vi "SendEmail.vi"(0 "To Address":string="kchambe1@nd.edu", 1 "To DisplayName":string="Karen Ostdiek ", 2 "Path to File":path=path "C:/Users/Public/Documents/AMS_VIs/2015/Karen/textfile", 3 "Subject":string, 4 "Body":string) -> ()   [LabVIEW 2014]
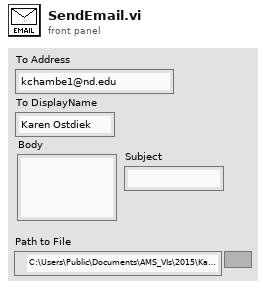
[diagram p1: front panel]
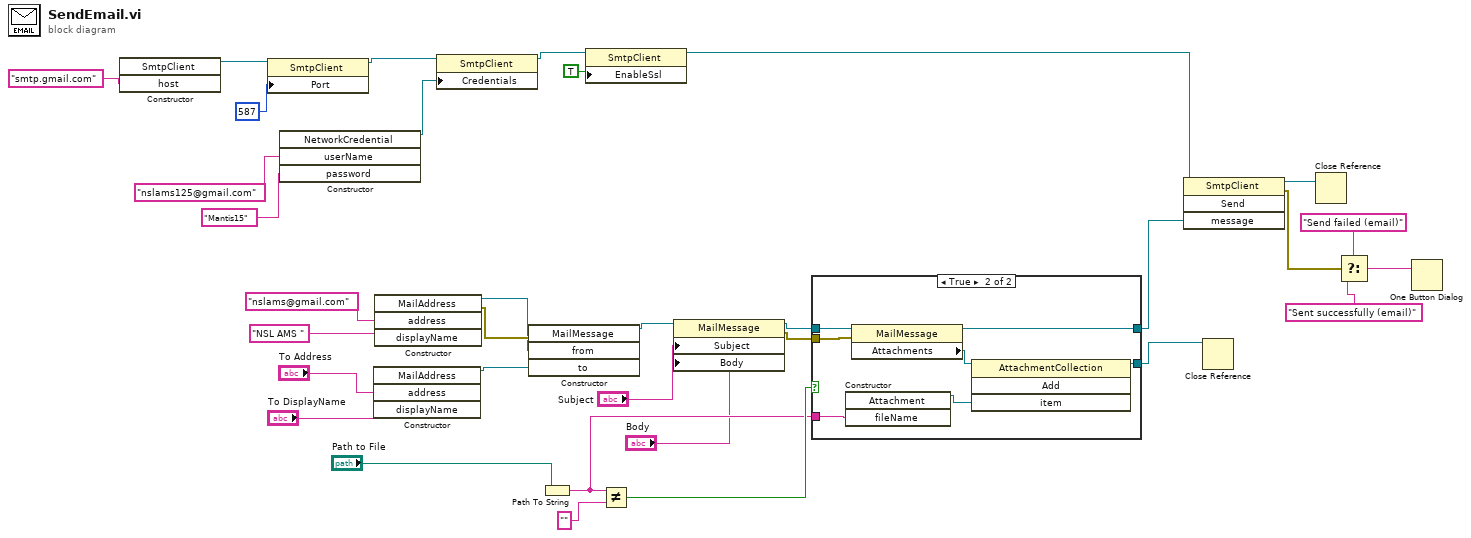
[diagram p0: block diagram]
diagram:
  n1 = constructor class="SmtpClient"("host"="smtp.gmail.com") -> (reference out=w32:refnum<k24>)  [unwired: 3 in, 3 out]
  n2 = property class="SmtpClient"(reference=w32, "Port"=587) -> (reference out=w30:refnum<k24>)  [unwired: 1 in, 1 out]
  n3 = constructor class="NetworkCredential"("userName"="nslams125@gmail.com", "password"="Mantis15") -> (reference out=w27:refnum<k24>)  [unwired: 3 in, 4 out]
  n4 = constructor class="MailAddress"("address"="To Address", "displayName"="To DisplayName") -> (reference out=w17:refnum<k24>)  [unwired: 3 in, 4 out]
  n5 = constructor class="MailAddress"("address"="nslams@gmail.com", "displayName"="NSL AMS ") -> (reference out=w18:refnum<k24>, error out=w19:errorcluster)  [unwired: 3 in, 3 out]
  n6 = property class="SmtpClient"(reference=w30, "Credentials"=w27) -> (reference out=w26:refnum<k24>)  [unwired: 1 in, 1 out]
  n7 = constructor class="MailMessage"(error in=w19, "from"=w18, "to"=w17) -> (reference out=w16:refnum<k24>)  [unwired: 2 in, 4 out]
  n8 = Path To String(path="Path to File") -> (string=w10:string)
  n9 = property class="SmtpClient"(reference=w26, "EnableSsl"=TRUE) -> (reference out=w25:refnum<k24>)  [unwired: 1 in, 1 out]
  n10 = Not Equal?(x=w10, y="") -> (x != y?=w13:bool)
  n11 = property class="MailMessage"(reference=w16, "Subject"="Subject", "Body"="Body") -> (reference out=w12:refnum<k24>, error out=w11:errorcluster)  [unwired: 1 in]
  n12 = case shown="True" w13 {
    tunnel: w12 -> [w34 w41]
    tunnel: w11 -> [_ w40]
    tunnel: w10 -> [_ w39]
    tunnel: [w34 w36] -> w9
    tunnel: [_ w35] -> w8
    frame False {
    }
    frame True {
      n13 = constructor class="Attachment"("fileName"=w39) -> (reference out=w37:refnum<k24>)  [unwired: 3 in, 3 out]
      n14 = property class="MailMessage"(reference=w41, error in=w40) -> (reference out=w36:refnum<k24>, "Attachments"=w38:refnum<k24>)  [unwired: 1 out]
      n15 = invoke class="AttachmentCollection" method="Add"(reference=w38, "item"=w37) -> (reference out=w35:refnum<k24>)  [unwired: 2 in, 3 out]
    }
  }
  n16 = invoke class="SmtpClient" method="Send"(reference=w25, "message"=w9) -> (reference out=w24:refnum<k24>, error out=w1:errorcluster)  [unwired: 2 in, 2 out]
  n17 = Close Reference(reference=w8) -> ()  [unwired: 1 in, 1 out]
  n18 = Close Reference(reference=w24) -> ()  [unwired: 1 in, 1 out]
  n19 = Select(t="Send failed (email)", s=w1, f="Sent successfully (email)") -> (s? t:f=w2:string)
  n20 = One Button Dialog(message=w2) -> ()  [unwired: 1 in, 1 out]
